vi "TSPopup.Close.vi"(8 "error in (no error)":errorcluster, 11 "TSPopup in":refnum<class "TSPopup.lvclass">) -> (0 "error out":errorcluster, 3 "TSPopup out":refnum<class "TSPopup.lvclass">)   [LabVIEW 2016, in "TSPopup.lvlib" / "TSPopup.lvclass"]
doc: "Closes the Type Sensitive Popup. Run at end of program.\n\nType Sensitive Popup \nCopyright © 2007, J. David Saunders\nAll rights reserved."
uses:
  <userlib>/TSPopup/TSPopup.lvclass
  <userlib>/TSPopup/TSPopup.lvclass/TSPopup.ctl
panel:
  # "Type Sensitive Popup \nCopyright © 2007, J. David Saunders\nAll rights reserved."
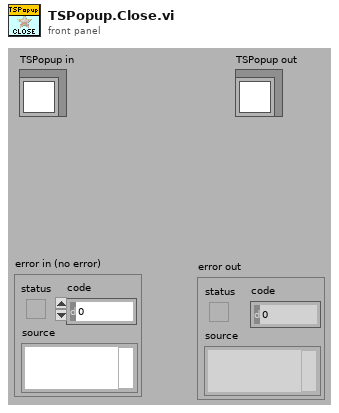
[diagram p1: front panel]
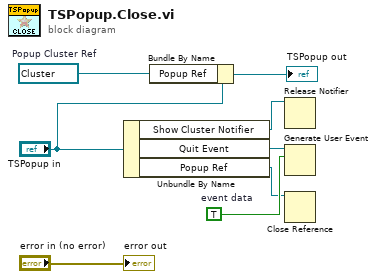
[diagram p0: block diagram]
diagram:
  w2 = refnum<vi> refnum  # Popup Cluster Ref
  w5 = TRUE  # event data
  n1 = Unbundle By Name("TSPopup in") -> ("Show Cluster Notifier"=w1:refnum<notifier>, "Quit Event"=w4:refnum<user-event>, "Popup Ref"=w3:refnum<vi>)
  n2 = Bundle By Name(cluster="TSPopup in", "Popup Ref"=w2) -> (→"TSPopup out":refnum<class "TSPopup.lvclass">)
  n3 = Release Notifier(notifier=w1) -> ()  [unwired: 2 in, 3 out]
  n4 = Generate User Event(user event=w4, event data cluster=w5) -> ()  [unwired: 2 in, 2 out]
  n5 = Close Reference(reference=w3) -> ()  [unwired: 1 in, 1 out]
  "error out" <- "error in (no error)"
